vi "SaveMovieFile_Array.vi"(6 "Formating":cluster{"Format":u16, "Compression":i32}={"Format"=0, "Compression"=1024} {"Compression" scale=0.0..1024.0 scale format="%.0x"; "Format" items=["Animation ' elr'", "Apple Intermediate Codec 'doci'", "Apple Pixlet Video 'tlxp'", "BMP 'ELRW'", "Cinepak 'divc'", "Component Video '2vuy'", "DV - PAL 'pcvd'", "DV/DVCPRO - NTSC ' cvd'", "DVCPRO - PAL 'ppvd'", "DVCPRO50 - NTSC 'n5vd'", "DVCPRO50 - PAL 'p5vd'", "Graphics ' cms'", "H.261 '162h'", "H.263 '362h'", "H.264 '1cva'", "JPEG 2000 '2pjm'", "Motion JPEG A 'apjm'", "Motion JPEG B 'bpjm'", "MPEG-4 Video 'v4pm'", "None ' war'", "Photo - JPEG 'gepj'", "Planar RGB 'SPB8'", "PNG ' gnp'", "Sorenson Video '1QVS'", "Sorenson Video 3 '3QVS'", "TGA ' agt'", "TIFF 'ffit'", "Video 'azpr'"]}, 8 "Frame duration [ms]":i32=200, 9 "Movie Settings":T2={"Width"=320, "Height"=240, "Time Base"=1000, "Type"=0, "Creator"=0, "Flatten"=0, "Options"=0, "Author"="Chris", "Information"="from LV Qt tlbx", "Copyright"="©94-2002", "Dialogs"=0} {"Dialogs" format="%.0b"}, 10 "Array of Images":T1[](array[typedef]) {"Dialogs" format="%.0b"}, 11 "Movie path":path) -> ()   [LabVIEW 2024]
doc: "Create a video movie made of LV images. The images can be compressed.\n\n© Chris Salzmann, 1994-2003"
uses:
  <userlib>/ImageProcessing/QTLIB_2595_LV86/QT_Private.ctl
  <userlib>/ImageProcessing/QTLIB_2595_LV86/QT_File.ctl
  <userlib>/ImageProcessing/QTLIB_2595_LV86/QT_Compression.ctl
  <userlib>/ImageProcessing/QTLIB_2595_LV86/QT_Movie.ctl
  <userlib>/ImageProcessing/QTLIB_2595_LV86/QT_Image.ctl
panel:
  out "Current Frame":picture
  out "error out":errorcluster={"status"=TRUE, "code"=-43, "source"=""}
  in  "stop":bool
  # "Create a video movie made of LV images. The images can be compressed.\n\n© Chris Salzmann, 1994-2005"
  # "Amination is lossless\nJPEG provides hight compression\nNo temporal compression at this time!"
  # "Min"
  # "Normal"
  # "Loss less"
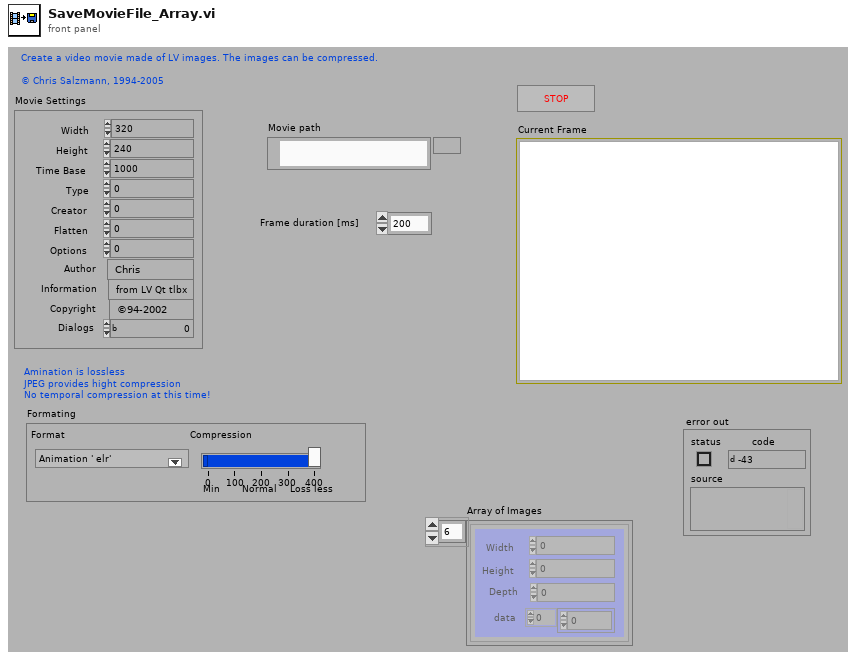
[diagram p1: front panel]
types:
  T1 = typedef "QT_Image.ctl" = cluster{"Width":i32, "Height":i32, "Depth":i32, "data":u8[], "Compressed data":u8[], "Color table":u32[], "Duration":i32, "Options":i32, "Timestamp":i32, "ID":i32, "Reserved":i32, "Dialogs":u32}
  T2 = typedef "QT_Movie.ctl" = cluster{"Width":i32, "Height":i32, "Time Base":i32, "Type":i32, "Creator":i32, "Flatten":i32, "Options":i32, "Author":string, "Information":string, "Copyright":string, "Dialogs":u32}
  T3 = typedef "QT_Compression.ctl" = cluster{"Compression":i32, "Format":i32, "Codec":i32, "Comp. Quality":i32, "Key Frame":i32, "Dialogs":u32}
  T4 = typedef "QT_File.ctl" = cluster{"Paths":string[], "Options":i32, "Dialogs":u32, "Reserved":i32}
  T5 = typedef "QT_Private.ctl" = cluster{"reserved 1":i32, "reserved 2":i32, "reserved 3":i32, "reserved 4":i32}
  T6 = typedef "QT_Ref.ctl" = refnum<k1>
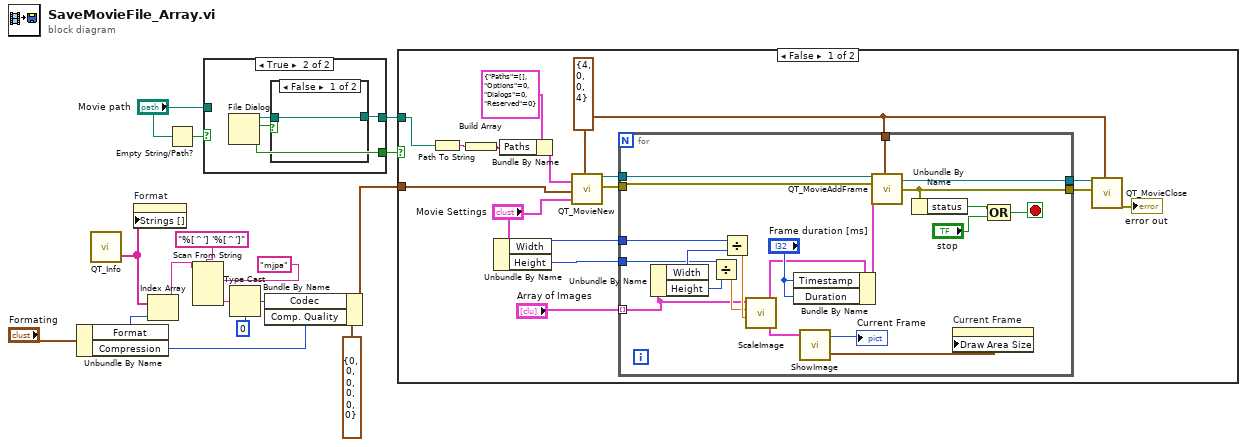
[diagram p0: block diagram]
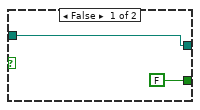
[diagram p3: hidden frame]
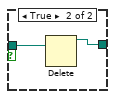
[diagram p4: hidden frame]
diagram:
  n1 = Unbundle By Name("Formating") -> ("Format"=w2:u16, "Compression"=w1:i32)
  n2 = call <userlib>:"QT_Info.vi"() -> ("Codec"=w11:string[])  [unwired: 3 in, 16 out]
  n3 = property on="Format" class="Ring (strict)"("Strings []"=w11) -> ()  [unwired: 2 in, 2 out]
  n4 = Index Array(array=w11, index=w2) -> (element=w10:string)
  n5 = Empty String/Path?(string/path="Movie path") -> (empty?=w7:bool)
  n6 = Scan From String(format string="%[^'] '%[^']", input string=w10) -> ()  [unwired: 2 in, 7 out]
  n7 = case shown="True" w7 {
    tunnel: [w17 w18] -> w6
    tunnel: [FALSE ("cancelled") w21] -> w5
    tunnel: "Movie path" -> [w17 _]
    frame False {
    }
    frame True {
      n8 = File Dialog() -> (1:w21:bool, 2:w20:bool, 3:w19:path)  [unwired: 1 in, 7 out]
      n9 = case shown="False" w20 {
        tunnel: w19 -> [w22 w24]
        tunnel: [w22 w23] -> w18
        frame False {
        }
        frame True {
          n10 = Delete(path (use dialog)=w24) -> (deleted path=w23:path)  [unwired: 4 in, 2 out]
        }
      }
    }
  }
  n11 = Type Cast(type=0 ("Format"), x="mjpa" ("format string")) -> (*(type *) &x=w15:i32)
  n12 = Bundle By Name(cluster=T3 {"Compression"=0, "Format"=0, "Codec"=0, "Comp. Quality"=0, "Key Frame"=0, "Dialogs"=0} ("Compression Settings"), "Codec"=w15, "Comp. Quality"=w1) -> (w12:T3)
  n13 = case shown="False" w5 {
    tunnel: w12 -> [w30 _]
    tunnel: w6 -> [w25 _]
    frame False {
      w35 = T5 {"reserved 1"=4, "reserved 2"=0, "reserved 3"=0, "reserved 4"=4} ("Private")
      n14 = Path To String(path=w25) -> (string=w40:string)
      n15 = Build Array(w40) -> (w29:string[])
      n16 = Unbundle By Name("Movie Settings") -> ("Width"=w27:i32, "Height"=w26:i32)
      n17 = Bundle By Name(cluster=T4 {"Paths"=[], "Options"=0, "Dialogs"=0, "Reserved"=0} ("File Settings"), "Paths"=w29) -> (w36:T4)
      n18 = call <userlib>:"QT_MovieNew.vi"("File Settings"=w36, "Movie Settings"="Movie Settings", "Compression Settings"=w30, "Private"=w35) -> ("QT Ref Out"=w38:T6, "error out"=w34:errorcluster)  [unwired: 2 in, 12 out]
      n19 = for {
        tunnel: [w55] -> w33
        tunnel: w34 -> [w57]
        tunnel: w35 -> [w58]
        tunnel: [w59] -> w39
        tunnel: w38 -> [w60]
        tunnel: "Array of Images" -> [w41] mode=indexing
        tunnel: w27 -> [w48]
        tunnel: w26 -> [w45]
        stop <- w51 stop-if-true
        n20 = Unbundle By Name(w41) -> ("Width"=w47:i32, "Height"=w44:i32)
        n21 = Divide(x=w45, y=w44) -> (x/y=w43:dbl)
        n22 = Divide(x=w48, y=w47) -> (x/y=w46:dbl)
        n23 = call <userlib>:"ScaleImage.vi"("X scale"=w46, "Y scale"=w43, "Image in"=w41) -> ("Image Out"=w50:T1)  [unwired: 2 in]
        n24 = Bundle By Name(cluster=w50, "Timestamp"="Frame duration [ms]", "Duration"="Frame duration [ms]") -> (w56:T1)
        n25 = call <userlib>:"ShowImage.vi"("Image"=w50) -> ("dimensions"=w42:cluster{"Witdh":i32, "Height":i32}, "image"=→"Current Frame":picture)  [unwired: 2 in]
        n26 = call <userlib>:"QT_MovieAddFrame.vi"("QT Ref In"=w60, "Image in"=w56, "error in (no error)"=w57, "Private"=w58) -> ("QT Ref Out"=w59:T6, "error out"=w55:errorcluster)  [unwired: 1 in, 13 out]
        n27 = Unbundle By Name(w55) -> ("status"=w54:bool)
        n28 = property on="Current Frame" class="Pict"("Draw Area Size"=w42) -> ()  [unwired: 2 in, 2 out]
        n29 = Compound Arithmetic op=OR(w54, "stop") -> (w51:bool)
      }
      n30 = call <userlib>:"QT_MovieClose.vi"("QT Ref In"=w39, "error in (no error)"=w33, "Private"=w35) -> ("error out"=→"error out":errorcluster)  [unwired: 16 out]
    }
    frame True {
    }
  }
